vi "get_keys_values.vi"(11 "Conditions":map{string, i32}(c390)) -> (2 "wartosci":i32[](array[numeric]), 3 "naglowki":string[](array[string]))   [LabVIEW 2019]
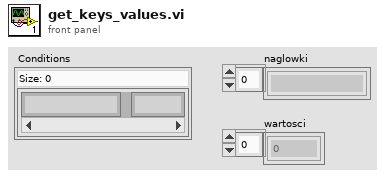
[diagram p1: front panel]
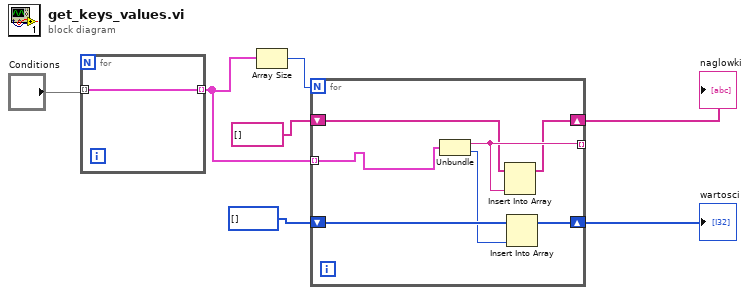
[diagram p0: block diagram]
diagram:
  n1 = for {
    tunnel: [w8] -> w3 mode=indexing
    tunnel: "Conditions" -> [w8] mode=indexing
  }
  n2 = Array Size(array=w3) -> (size(s)=w5:i32)
  n3 = for {
    N: w5 -> [_]
    tunnel: w3 -> [w15] mode=indexing
    tunnel: [w14] -> _ mode=indexing
    shift-right: [w12] -> w6
    shift-left: string[] [] ("array") -> [w13]
    shift-right: [w10] -> w7
    shift-left: i32[] [] ("array") -> [w11]
    n4 = Unbundle(w15) -> (w14:string, w9:i32)
    n5 = Insert Into Array(array=w13, new element=w14) -> (w12:string[])  [unwired: 1 in]
    n6 = Insert Into Array(array=w11, new element=w9) -> (w10:i32[])  [unwired: 1 in]
  }
  "wartosci" <- w7
  "naglowki" <- w6
